vi "Teleop.vi"(10 "Match Info":T1={"Autonomous Elapsed Seconds"=0.0, "TeleOp Elapsed Seconds"=0.0, "Disabled Elapsed Seconds"=0.0, "Visited Autonomous"=FALSE, "Visited TeleOp"=FALSE, "Visited Disabled"=FALSE, "Autonomous Settings"={"Autonomous Style"=enum."Independent", "VI Refnum"=refnum}}, 11 "Call Context":T2) -> ()   [LabVIEW 2015]
doc: "This VI is called for each TeleOp packet received from the DS where the robot is not disabled. It is often used to read from the joysticks and update I/O or to update setpoints for timed control loops. It should complete and return within 20 milliseconds or it may miss DS packets."
uses:
  <vilib>/Rock Robotics/WPI/DriverStation/WPI_DriverStationDerivedRobotMode.ctl
  <vilib>/Rock Robotics/WPI/DriverStation/WPI_DriverStationMatch Info.ctl
  <vilib>/Rock Robotics/WPI/Utilities/WPI_GetSetVariantRefNum.vi
  Robot Global Data.vi
  <vilib>/Rock Robotics/Network Tables/SD Write Number.vi
  <vilib>/Rock Robotics/WPI/Solenoid/Deprecated/WPI_SolenoidSetBool.vi
  <vilib>/Rock Robotics/Network Tables/NT Write Number.vi
  <vilib>/Rock Robotics/Network Tables/NT Write Boolean.vi
  Z navX/navX Library v2/navX Library v2.lvlib
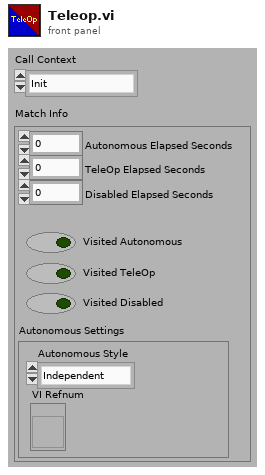
[diagram p1: front panel]
types:
  T1 = typedef "WPI_DriverStationMatch Info.ctl" = cluster{"Autonomous Elapsed Seconds":dbl, "TeleOp Elapsed Seconds":dbl, "Disabled Elapsed Seconds":dbl, "Visited Autonomous":bool, "Visited TeleOp":bool, "Visited Disabled":bool, "Autonomous Settings":cluster{"Autonomous Style":enum16{"Iterative", "Independent"}, "VI Refnum":refnum<vi>}}
  T2 = typedef "WPI_DriverStationDerivedRobotMode.ctl" = enum16{"Init", "Execute", "Stop"}
  T3 = enum16{"No Override", "Override to Coast", "Override to Brake"}
  T4 = typedef "WPI_JoystickDevRef.ctl" = cluster{"Device":T5}
  T5 = typedef "WPI_JoystickDeviceEnum.ctl" = enum16{"USB 0", "USB 1", "USB 2", "USB 3", "USB 4", "USB 5"}
  T6 = cluster{"Axes[0]":dbl, "Axes[1]":dbl, "Axes[2]":dbl, "Axes[3]":dbl, "Axes[4]":dbl, "Axes[5]":dbl, "Axes[6]":dbl, "Axes[7]":dbl, "Axes[8]":dbl}
  T7 = cluster{"Buttons[0]":bool, "Buttons[1]":bool, "Buttons[2]":bool, "Buttons[3]":bool, "Buttons[4]":bool, "Buttons[5]":bool, "Buttons[6]":bool, "Buttons[7]":bool, "Buttons[8]":bool}
  T8 = typedef "navX Library v2.lvlib/Z900_navX_DeviceTypeDef.ctl" = cluster{"Interface":cluster{"Protocol":T9, "Update Rate (4Hz-60Hz)":u8, "navX Open TypeDef":variant}, "Notify Packet":refnum<notifier>, "Loop VI Refnum":refnum<vi>, "Ready to Close Occurrence Refnum":refnum<k4>}
  T9 = typedef "navX Library v2.lvlib/Z900_navX_ProtocolTypeDef.ctl" = enum16{"SERIAL", "I2C", "SPI"}
  T10 = cluster{"Yaw":dbl, "Roll":dbl, "Pitch":dbl, "Heading":dbl, "Fused Heading":dbl}
  T11 = cluster{"LinearAcceleration X":dbl, "LinearAcceleration Y":dbl, "LinearAcceleration Z":dbl}
  T12 = cluster{"Velocity X":dbl, "Velocity Y":dbl, "Velocity Z":dbl, "Displacement X":dbl, "Displacement Y":dbl, "Displacement Z":dbl}
  T13 = typedef "WPI_MotorControlDeviceRef.ctl" = cluster{"DeviceStatus":errorcluster, "Type":T14, "PWM":cluster{"PWM Channel":T15, "DeadBand":T16}, "CAN":cluster{"Device Number":u8, "Control Mode":T17, "Semaphore":T18, "Max Vout":dbl, "TalonSRX Control Mode":T19}, "Invert":bool}
  T14 = typedef "WPI_MotorControlType.ctl" = enum16{"PWM", "CAN", "CANTalonSRX"}
  T15 = typedef "FPGA_DIOPWMChannel.ctl" = enum8{"PWM 0", "PWM 1", "PWM 2", "PWM 3", "PWM 4", "PWM 5", "PWM 6", "PWM 7", "PWM 8", "PWM 9", "PWM MXP 0", "PWM MXP 1", "PWM MXP 2", "PWM MXP 3", "PWM MXP 4", "PWM MXP 5", "PWM MXP 6", "PWM MXP 7", "PWM MXP 8", "PWM MXP 9", "Invalid"}
  T16 = typedef "WPI_PWMDeadband.ctl" = cluster{"Name":string, "maxPositivePwm":i32, "minPositivePwm":i32, "centerPwm":i32, "maxNegativePwm":i32, "minNegativePwm":i32, "angularRange":u16}
  T17 = typedef "WPI_CANJaguar_ControlMode.ctl" = enum8{"Percent VBus", "Current", "Speed", "Position", "Voltage"}
  T18 = typedef "Semaphore RefNum" = refnum<k1>
  T19 = typedef "WPI_CANTalonSRX_APIControlMode.ctl" = enum8{"Percent VBus", "Speed", "Position", "Slave", "Unchanged / Invalid", "Voltage Compensation", "Current", "Motion Profile"}
  T20 = typedef "WPI_SolenoidDevRef.ctl" = cluster{"DevStatus":errorcluster, "Pneumatics Control Module":u8, "Forward Solenoid Channel":T21, "Reverse Solenoid Channel":T21}
  T21 = typedef "WPI_SolenoidChannel.ctl" = enum8{"Solenoid 0", "Solenoid 1", "Solenoid 2", "Solenoid 3", "Solenoid 4", "Solenoid 5", "Solenoid 6", "Solenoid 7", "Invalid"}
  T22 = typedef "WPI_CANTalonSRX_GlobalStatus.ctl" = cluster{"Applied Throttle":dbl, "Module Enabled":bool, "CAN Error":errorcluster, "Closed Loop Error":dbl, "Forward Limit Switch Closed":bool, "Reverse Limit Switch Closed":bool, "Sensor Position":dbl, "Sensor Velocity":dbl, "Current":dbl, "Sticky Fault - Over Temp":bool, "Sticky Fault - Under Voltage":bool, "Sticky Fault - Forward Limit":bool, "Sticky Fault - Reverse Limit":bool, "Sticky Fault - Forward Soft Limit":bool, "Sticky Fault - Reverse Soft Limit":bool, "Brake is Enabled":bool, "Encoder Position":dbl, "Encoder Velocity":dbl, "Encoder Index Count":dbl, "Encoder A Pin State":bool, "Encoder B Pin State":bool, "Encoder Index Pin State":bool, "Analog In":dbl, "Analog In Velocity":dbl, "Temperature (C)":dbl, "Battery Voltage":dbl, "Control 5 Is Supported":bool, "Current Profile Slot Select":dbl, "Pos Div 8":bool, "Vel Div 4":bool, "Pulse Width Position":i32, "Pulse Width Velocity":i32, "Pulse Width Rise To Rise (us)":i32, "Pulse Width Rise To Fall (us)":i32, "Mot Prof Active Is Under Run":bool, "Mot Prof Active Has Under Run":bool, "Mot Prof Active Is Last":bool, "Mot Prof Active Velocity Only":bool, "Mot Prof Active Is Valid":bool, "Mot Prof Buffer Is Full":bool, "Mot Prof Active Profile Slot Select":i32, "Mot Prof NextID":i32, "Mot Prof Count":i32, "Mot Prof Active Velocity":dbl, "Mot Prof Active Position":dbl, "Mot Prof Output Enable":i32}
  T23 = typedef "WPI_RobotDriveDevRef.ctl" = cluster{"DevStatus":errorcluster, "Motors[]":T13[], "Square Inputs":bool, "Max Output":dbl}
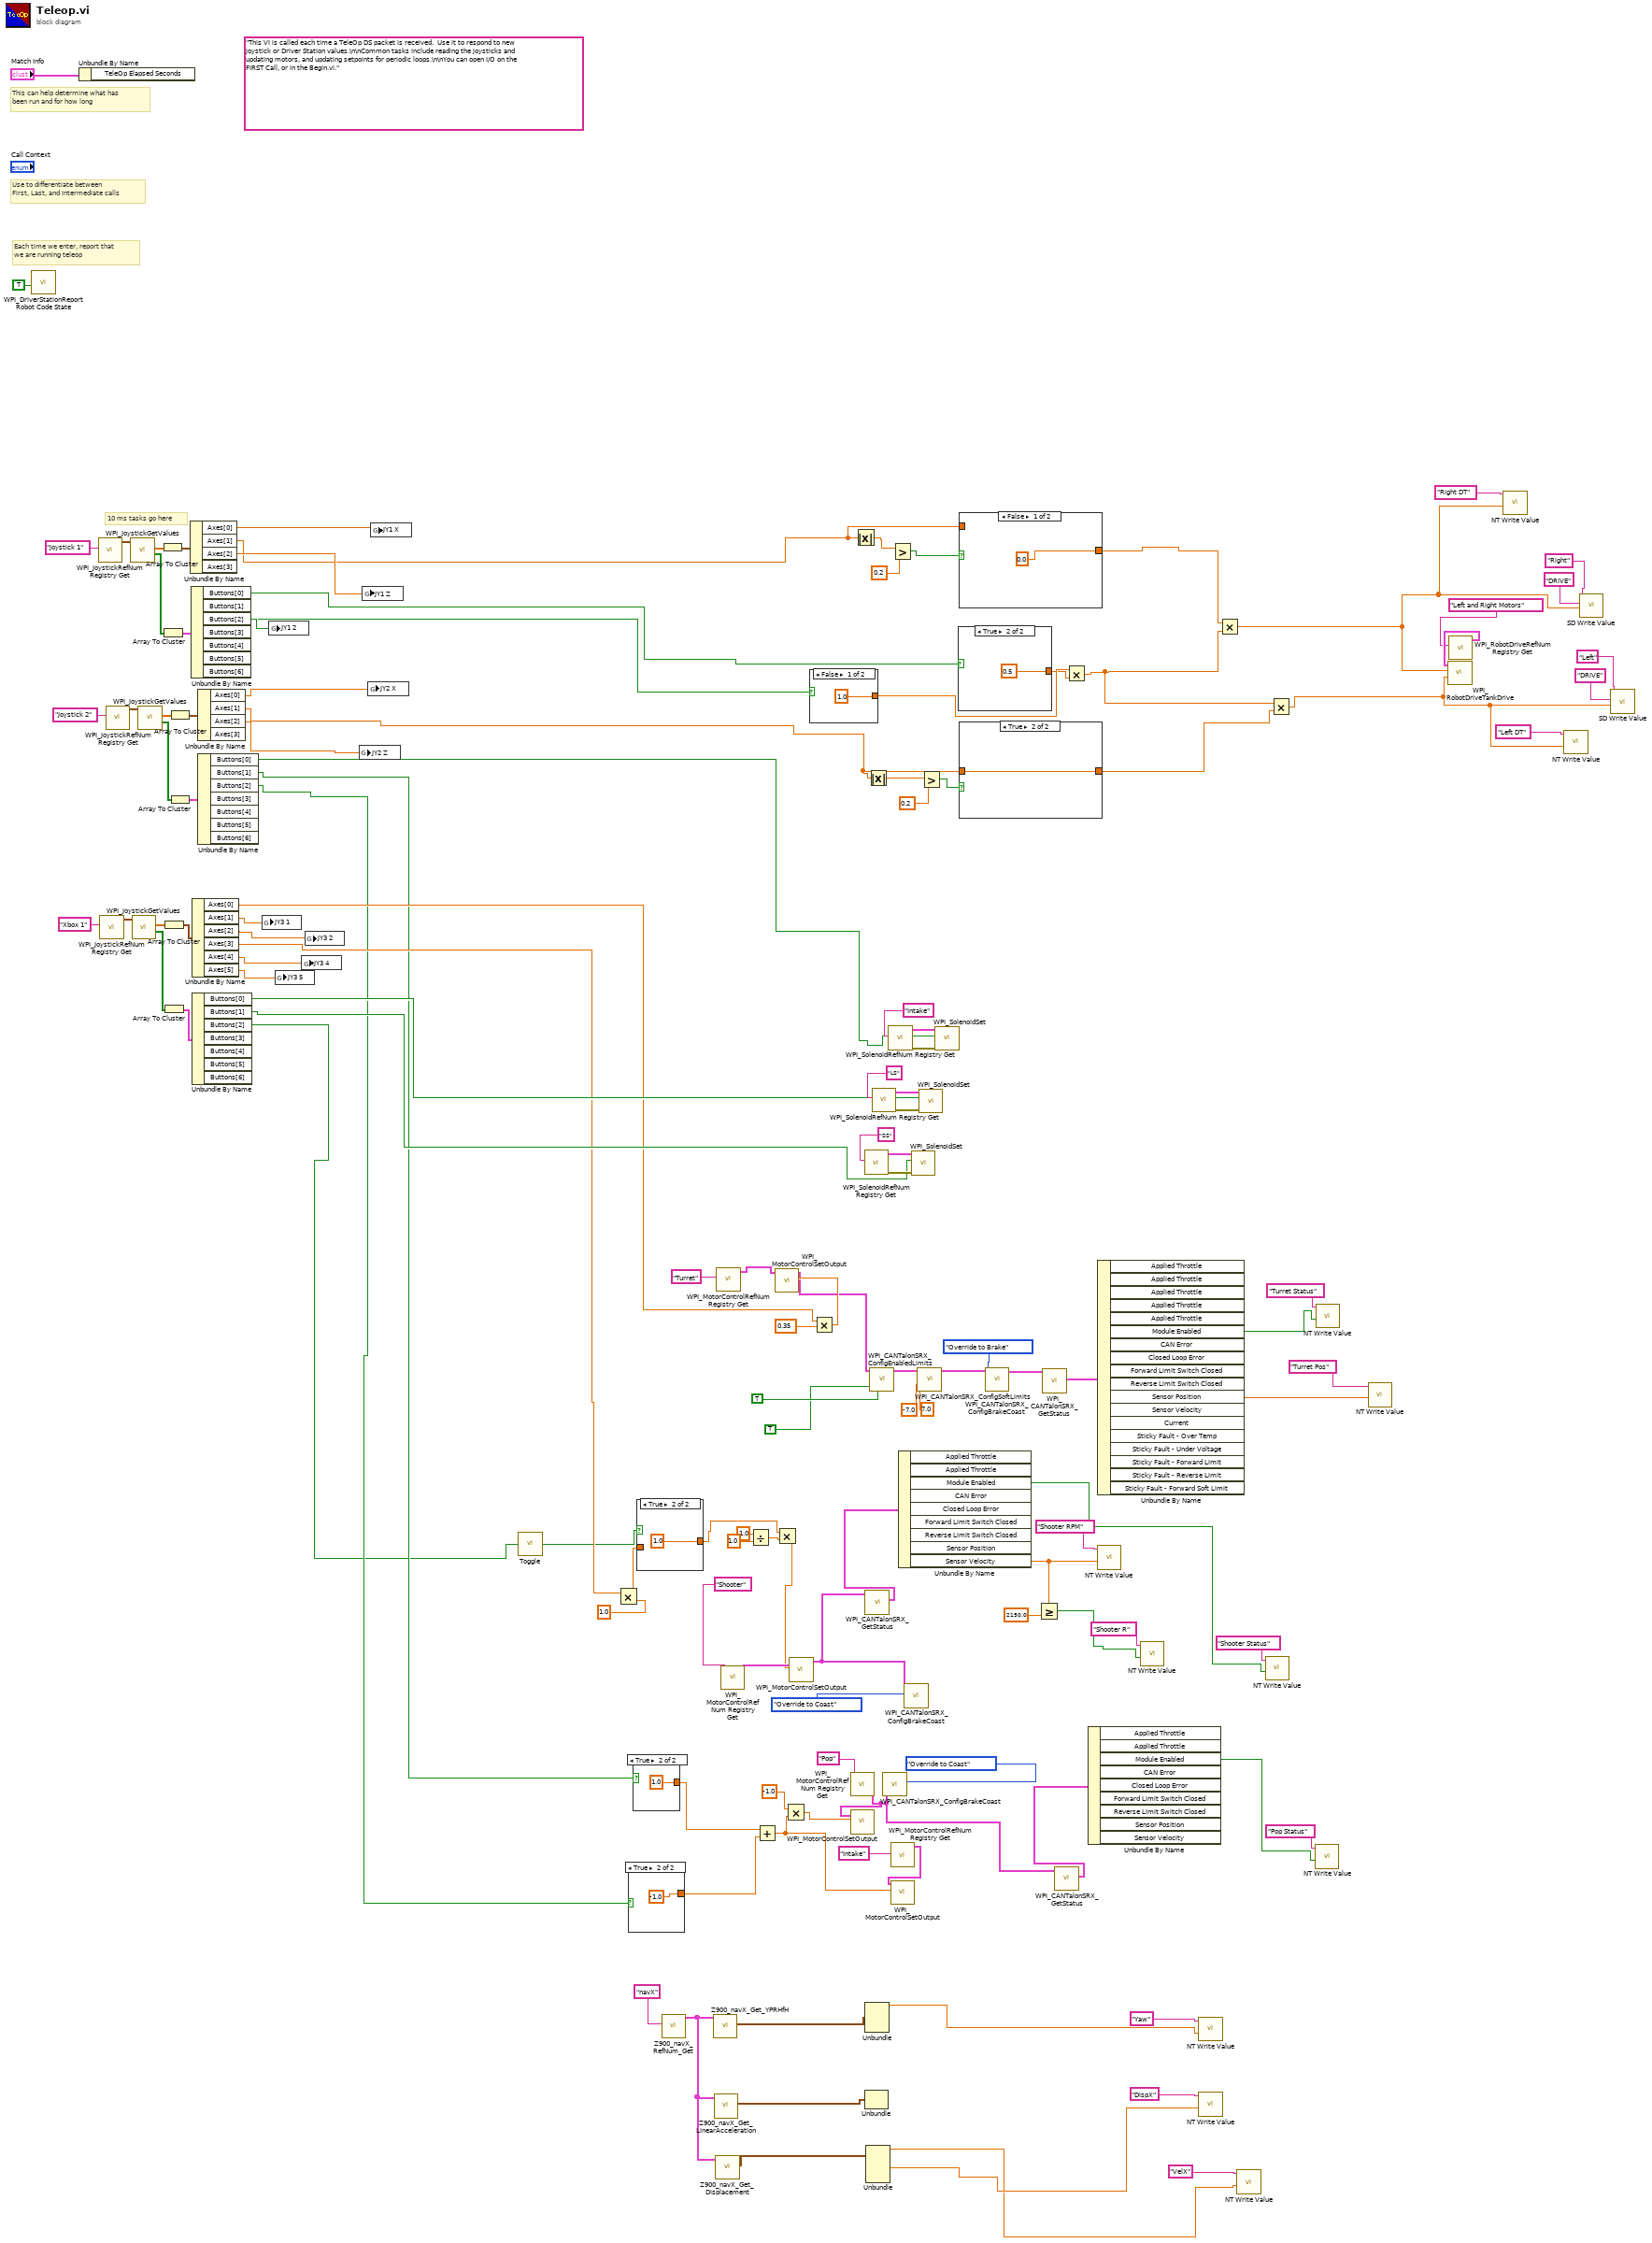
[diagram p0: block diagram]
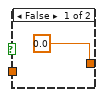
[diagram p2: hidden frame]
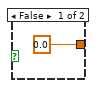
[diagram p3: hidden frame]
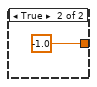
[diagram p4: hidden frame]
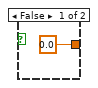
[diagram p5: hidden frame]
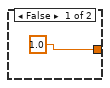
[diagram p6: hidden frame]
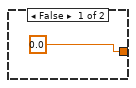
[diagram p7: hidden frame]
diagram:
  (unwired) "This VI is called each time a TeleOp DS packet is received.  Use it to respond to new joystick or Driver Station values.\n\nCommon tasks include reading the joysticks and updating motors, and updating setpoints for periodic loops.\n\nYou can open I/O on the FIRST Call, or in the Begin.vi."
  # "10 ms tasks go here"
  # "Each time we enter, report that\nwe are running teleop"
  # "Use to differentiate between\nFirst, Last, and Intermediate calls"
  # "This can help determine what has\nbeen run and for how long"
  n1 = call <vilib>:"WPI_DriverStationReport Robot Code State.vi"("TeleOp"=TRUE ("Autonomous")) -> ()  [unwired: 10 in, 1 out]
  n2 = Unbundle By Name("Match Info") -> ()  [unwired: 1 out]
  n3 = call <vilib>:"WPI_JoystickRefNum Registry Get.vi"("refnum name"="Joystick 1") -> ("JoystickDevRef"=w88:T4)  [unwired: 1 in, 9 out]
  n4 = call <vilib>:"WPI_JoystickRefNum Registry Get.vi"("refnum name"="Xbox 1") -> ("JoystickDevRef"=w76:T4)  [unwired: 1 in, 9 out]
  n5 = call <vilib>:"WPI_JoystickRefNum Registry Get.vi"("refnum name"="Joystick 2") -> ("JoystickDevRef"=w82:T4)  [unwired: 1 in, 9 out]
  n6 = call <vilib>:"WPI_JoystickGetValues.vi"("JoystickDevRef"=w88) -> ("Buttons"=w86:bool[], "Axes"=w85:dbl[])  [unwired: 6 in, 3 out]
  n7 = call <vilib>:"WPI_JoystickGetValues.vi"("JoystickDevRef"=w76) -> ("Buttons"=w74:bool[], "Axes"=w73:dbl[])  [unwired: 6 in, 3 out]
  n8 = call <vilib>:"WPI_JoystickGetValues.vi"("JoystickDevRef"=w82) -> ("Buttons"=w80:bool[], "Axes"=w79:dbl[])  [unwired: 6 in, 3 out]
  n9 = Array To Cluster(array=w85) -> (cluster=w87:T6)
  n10 = Array To Cluster(array=w86) -> (cluster=w84:T7)
  n11 = Array To Cluster(array=w73) -> (cluster=w75:T6)
  n12 = Array To Cluster(array=w74) -> (cluster=w72:T7)
  n13 = Array To Cluster(array=w79) -> (cluster=w81:T6)
  n14 = Array To Cluster(array=w80) -> (cluster=w78:T7)
  n15 = Unbundle By Name(w87) -> ("Axes[0]"=w70:dbl, "Axes[1]"=w60:dbl, "Axes[2]"=w69:dbl)  [unwired: 1 out]
  n16 = Unbundle By Name(w84) -> ("Buttons[0]"=w62:bool, "Buttons[1]"=w61:bool, "Buttons[2]"=w63:bool)  [unwired: 4 out]
  n17 = Unbundle By Name(w75) -> ("Axes[0]"=w42:dbl, "Axes[1]"=w66:dbl, "Axes[2]"=w64:dbl, "Axes[3]"=w51:dbl, "Axes[4]"=w65:dbl, "Axes[5]"=w71:dbl)
  n18 = Unbundle By Name(w72) -> ("Buttons[0]"=w57:bool, "Buttons[1]"=w56:bool, "Buttons[2]"=w11:bool)  [unwired: 4 out]
  n19 = Unbundle By Name(w81) -> ("Axes[0]"=w68:dbl, "Axes[1]"=w59:dbl, "Axes[2]"=w67:dbl)  [unwired: 1 out]
  n20 = Unbundle By Name(w78) -> ("Buttons[0]"=w58:bool, "Buttons[1]"=w35:bool, "Buttons[2]"=w34:bool)  [unwired: 4 out]
  n21 = global write "Robot Global Data.vi" "JY3 1"(w66) -> ()
  n22 = global write "Robot Global Data.vi" "JY1 2"(w63) -> ()
  n23 = global write "Robot Global Data.vi" "JY3 5"(w71) -> ()
  n24 = global write "Robot Global Data.vi" "JY3 4"(w65) -> ()
  n25 = global write "Robot Global Data.vi" "JY3 2"(w64) -> ()
  n26 = global write "Robot Global Data.vi" "JY2 Z"(w67) -> ()
  n27 = global write "Robot Global Data.vi" "JY1 Z"(w69) -> ()
  n28 = global write "Robot Global Data.vi" "JY2 X"(w68) -> ()
  n29 = global write "Robot Global Data.vi" "JY1 X"(w70) -> ()
  n30 = call "Toggle.vi"("Input"=w11) -> ("Output"=w10:bool)
  n31 = Multiply(x=w51, y=1.0) -> (x*y=w12:dbl)
  n32 = case shown="True" w34 {
    tunnel: [0.0 -1.0] -> w100
    frame False {
    }
    frame True {
    }
  }
  n33 = case shown="True" w35 {
    tunnel: [0.0 1.0] -> w101
    frame False {
    }
    frame True {
    }
  }
  n34 = case shown="True" w10 {
    tunnel: w12 -> [_ _]
    tunnel: [0.0 1.0] -> w5
    frame False {
    }
    frame True {
    }
  }
  n35 = call "Z900_navX_RefNum_Get.vi"("refnum name"="navX") -> ("navX Device"=w54:T8)  [unwired: 9 in, 1 out]
  n36 = call "Z900_navX_Get_YPRHfH.vi"("navX Device"=w54) -> ("YRPHfH"=w55:T10)  [unwired: 7 in, 3 out]
  n37 = call "Z900_navX_Get_LinearAcceleration.vi"("navX Device"=w54) -> ("Linear Acceleration"=w53:T11)  [unwired: 7 in, 3 out]
  n38 = call "Z900_navX_Get_Displacement.vi"("navX Device"=w54) -> ("Displacement"=w52:T12)  [unwired: 7 in, 3 out]
  n39 = call <vilib>:"WPI_MotorControlRefNum Registry Get.vi"("refnum name"="Turret") -> ("MotorControlDevRef"=w41:T13)  [unwired: 9 in, 1 out]
  n40 = call <vilib>:"WPI_MotorControlRefNum Registry Get.vi"("refnum name"="Shooter") -> ("MotorControlDevRef"=w97:T13)  [unwired: 9 in, 1 out]
  n41 = Divide(x=1.0, y=1.0) -> (x/y=w7:dbl)
  n42 = Add(x=w101, y=w100) -> (x+y=w95:dbl)
  n43 = Multiply(x=w5, y=w7) -> (x*y=w6:dbl)
  n44 = Multiply(x=-1.0, y=w95) -> (x*y=w96:dbl)
  n45 = call <vilib>:"WPI_MotorControlSetOutput.vi"("Output"=w6, "MotorControlDevRef"=w97) -> ("MotorControlDevRef"=w92:T13)  [unwired: 7 in, 2 out]
  n46 = case shown="False" w61 {
    tunnel: [1.0 -1.0] -> w106
    frame False {
    }
    frame True {
    }
  }
  n47 = Multiply(x=w42, y=0.35) -> (x*y=w49:dbl)
  n48 = call <vilib>:"WPI_MotorControlSetOutput.vi"("Output"=w49, "MotorControlDevRef"=w41) -> ("MotorControlDevRef"=w40:T13)  [unwired: 7 in, 2 out]
  n49 = call <vilib>:"WPI_MotorControlRefNum Registry Get.vi"("refnum name"="Pop") -> ("MotorControlDevRef"=w15:T13)  [unwired: 9 in, 1 out]
  n50 = call <vilib>:"WPI_MotorControlSetOutput.vi"("Output"=w96, "MotorControlDevRef"=w15) -> ()  [unwired: 7 in, 3 out]
  n51 = Absolute Value(x=w60) -> (abs(x)=w127:dbl)
  n52 = call <vilib>:"WPI_SolenoidRefNum Registry Get.vi"("refnum name"="SS") -> ("error out"=w113:errorcluster, "SolenoidDevRef"=w114:T20)  [unwired: 9 in]
  n53 = Unbundle(w53) -> ()  [unwired: 3 out]
  n54 = call <vilib>:"WPI_CANTalonSRX_GetStatus.vi"("CAN Talon SRX Ref"=w92) -> ("Talon SRX Status"=w98:T22)  [unwired: 8 in, 2 out]
  n55 = Unbundle(w55) -> ("Yaw"=w22:dbl)  [unwired: 4 out]
  n56 = Unbundle(w52) -> ("Velocity X"=w20:dbl, "Displacement X"=w24:dbl)  [unwired: 4 out]
  n57 = Absolute Value(x=w59) -> (abs(x)=w126:dbl)
  n58 = call <vilib>:"WPI_CANTalonSRX_ConfigEnabledLimits.vi"("CAN Talon SRX Ref"=w40, "Forward Soft Limit Enable"=TRUE, "Reverse Soft Limit Enable"=TRUE) -> ("CAN Talon SRX Ref"=w39:T13)  [unwired: 11 in, 1 out]
  n59 = call <vilib>:"WPI_SolenoidRefNum Registry Get.vi"("refnum name"="LS") -> ("error out"=w116:errorcluster, "SolenoidDevRef"=w117:T20)  [unwired: 9 in]
  n60 = call <vilib>:"WPI_CANTalonSRX_ConfigBrakeCoast.vi"("Brake / Coast Mode"=T3."Override to Coast", "CAN Talon SRX Ref"=w15) -> ()  [unwired: 8 in, 2 out]
  n61 = call <vilib>:"WPI_SolenoidRefNum Registry Get.vi"("refnum name"="Intake") -> ("error out"=w110:errorcluster, "SolenoidDevRef"=w111:T20)  [unwired: 9 in]
  n62 = Greater?(x=w127, y=0.2) -> (0:w131:bool)
  n63 = call <vilib>:"WPI_MotorControlRefNum Registry Get.vi"("refnum name"="Intake") -> ("MotorControlDevRef"=w102:T13)  [unwired: 9 in, 1 out]
  n64 = call <vilib>:"WPI_MotorControlSetOutput.vi"("Output"=w95, "MotorControlDevRef"=w102) -> ()  [unwired: 7 in, 3 out]
  n65 = Unbundle By Name(w98) -> ("Module Enabled"=w18:bool, "Sensor Velocity"=w3:dbl)  [unwired: 7 out]
  n66 = call <vilib>:"WPI_CANTalonSRX_ConfigBrakeCoast.vi"("Brake / Coast Mode"=T3."Override to Coast", "CAN Talon SRX Ref"=w92) -> ()  [unwired: 8 in, 2 out]
  n67 = call-poly <vilib>:"WPI_SolenoidSet.vi"("error in (no error)"=w113, "Value"=w56, "SolenoidDevRef"=w114) -> ()  [unwired: 9 out]
  n68 = call <vilib>:"WPI_CANTalonSRX_ConfigSoftLimits.vi"("CAN Talon SRX Ref"=w39, "Forward Limit Position"=7.0, "Reverse Limit Position"=-7.0) -> ("CAN Talon SRX Ref"=w38:T13)  [unwired: 11 in, 1 out]
  n69 = call-poly <vilib>:"WPI_SolenoidSet.vi"("error in (no error)"=w116, "Value"=w57, "SolenoidDevRef"=w117) -> ()  [unwired: 9 out]
  n70 = Greater?(x=w126, y=0.2) -> (0:w129:bool)
  n71 = call-poly <vilib>:"WPI_SolenoidSet.vi"("error in (no error)"=w110, "Value"=w58, "SolenoidDevRef"=w111) -> ()  [unwired: 9 out]
  n72 = case shown="True" w62 {
    tunnel: [1.0 0.5] -> w104
    frame False {
    }
    frame True {
    }
  }
  n73 = case shown="False" w131 {
    tunnel: [0.0 w145] -> w120
    tunnel: w60 -> [_ w145]
    frame False {
    }
    frame True {
    }
  }
  n74 = case shown="True" w129 {
    tunnel: [0.0 w147] -> w121
    tunnel: w59 -> [_ _]
    tunnel: w59 -> [_ w147]
    frame False {
    }
    frame True {
    }
  }
  n75 = call <vilib>:"WPI_CANTalonSRX_ConfigBrakeCoast.vi"("Brake / Coast Mode"=T3."Override to Brake", "CAN Talon SRX Ref"=w38) -> ("CAN Talon SRX Ref"=w37:T13)  [unwired: 8 in, 1 out]
  n76 = Greater Or Equal?(x=w3, y=2150.0) -> (x >= y?=w1:bool)
  n77 = call <vilib>:"WPI_CANTalonSRX_GetStatus.vi"("CAN Talon SRX Ref"=w37) -> ("Talon SRX Status"=w36:T22)  [unwired: 8 in, 2 out]
  n78 = call <vilib>:"WPI_CANTalonSRX_GetStatus.vi"("CAN Talon SRX Ref"=w15) -> ("Talon SRX Status"=w16:T22)  [unwired: 8 in, 2 out]
  n79 = Multiply(x=w106, y=w104) -> (x*y=w105:dbl)
  n80 = Unbundle By Name(w16) -> ("Module Enabled"=w14:bool)  [unwired: 8 out]
  n81 = call-poly <vilib>:"NT Write Value.vi"("Numeric"=w3, "Name"="Shooter RPM") -> ()  [unwired: 9 in, 1 out]
  n82 = Unbundle By Name(w36) -> ("Module Enabled"=w30:bool, "Sensor Position"=w33:dbl)  [unwired: 16 out]
  n83 = call-poly <vilib>:"NT Write Value.vi"("Boolean"=w1, "Name"="Shooter R") -> ()  [unwired: 9 in, 1 out]
  n84 = call-poly <vilib>:"NT Write Value.vi"("Numeric"=w22, "Name"="Yaw") -> ()  [unwired: 9 in, 1 out]
  n85 = call-poly <vilib>:"NT Write Value.vi"("Numeric"=w24, "Name"="DispX") -> ()  [unwired: 9 in, 1 out]
  n86 = Multiply(x=w120, y=w105) -> (x*y=w26:dbl)
  n87 = call-poly <vilib>:"NT Write Value.vi"("Numeric"=w20, "Name"="VelX") -> ()  [unwired: 9 in, 1 out]
  n88 = call-poly <vilib>:"NT Write Value.vi"("Boolean"=w18, "Name"="Shooter Status") -> ()  [unwired: 9 in, 1 out]
  n89 = Multiply(x=w105, y=w121) -> (x*y=w28:dbl)
  n90 = call-poly <vilib>:"NT Write Value.vi"("Boolean"=w14, "Name"="Pop Status") -> ()  [unwired: 9 in, 1 out]
  n91 = call-poly <vilib>:"NT Write Value.vi"("Boolean"=w30, "Name"="Turret Status") -> ()  [unwired: 9 in, 1 out]
  n92 = call-poly <vilib>:"NT Write Value.vi"("Numeric"=w33, "Name"="Turret Pos") -> ()  [unwired: 9 in, 1 out]
  n93 = call <vilib>:"WPI_RobotDriveRefNum Registry Get.vi"("refnum name"="Left and Right Motors") -> ("RobotDriveDevRef"=w119:T23)  [unwired: 9 in, 1 out]
  n94 = call <vilib>:"WPI_RobotDriveTankDrive.vi"("Right axis value"=w28, "Left axis value"=w26, "RobotDriveDevRef"=w119) -> ()  [unwired: 6 in, 3 out]
  n95 = call-poly <vilib>:"NT Write Value.vi"("Numeric"=w26, "Name"="Right DT") -> ()  [unwired: 9 in, 1 out]
  n96 = call-poly <vilib>:"NT Write Value.vi"("Numeric"=w28, "Name"="Left DT") -> ()  [unwired: 9 in, 1 out]
  n97 = call-poly <vilib>:"SD Write Value.vi"("Numeric"=w26, "Table Prefix"="DRIVE", "Name"="Right") -> ()  [unwired: 7 in, 2 out]
  n98 = call-poly <vilib>:"SD Write Value.vi"("Numeric"=w28, "Table Prefix"="DRIVE", "Name"="Left") -> ()  [unwired: 7 in, 2 out]
